vi "MagPowSup.vi"() -> ()   [LabVIEW 2016]
uses:
  <vilib>/Math Plots/3D Math Plots/3D Comet/3D Comet Datatype/3D Comet Datatype.lvclass
  <vilib>/Math Plots/3D Math Plots/3D Comet/3D Comet Datatype/Public/Plot Helper (Vector).vi
  <vilib>/Math Plots/3D Math Plots/3D Comet/3D Comet XCtrl/3D Comet.xctl
panel:
  out "3D Comet":refnum<class "3D Plot Datatype.lvclass">[](xcontrol)
  in  "Z VISA In":refnum<visa-resource-name>="COM3"
  in  "Y VISA In":refnum<visa-resource-name>="COM3"
  out "Z VISA Out":refnum<visa-resource-name>
  out "Y VISA Out":refnum<visa-resource-name>
  out "X VISA Out":refnum<visa-resource-name>
  in  "X VISA In":refnum<visa-resource-name>="COM3"
  in  "Loop":bool
  in  "Loop":bool
  in  "Queue Z":string[][](table)
  in  "Queue Y":string[][](table)
  in  "Queue X":string[][](table)
  in  "Loop":bool
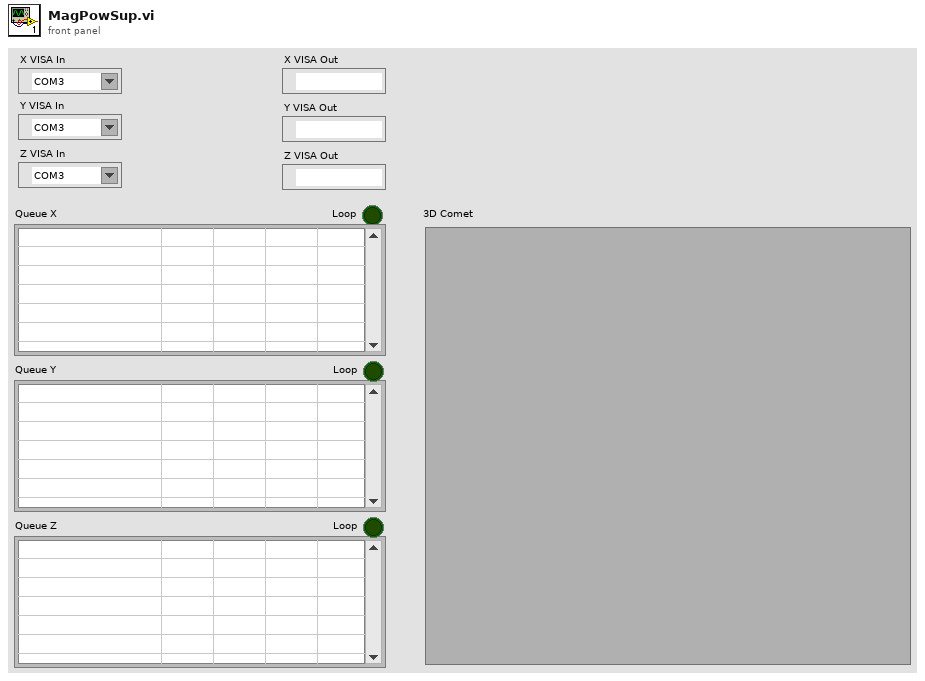
[diagram p1: front panel]
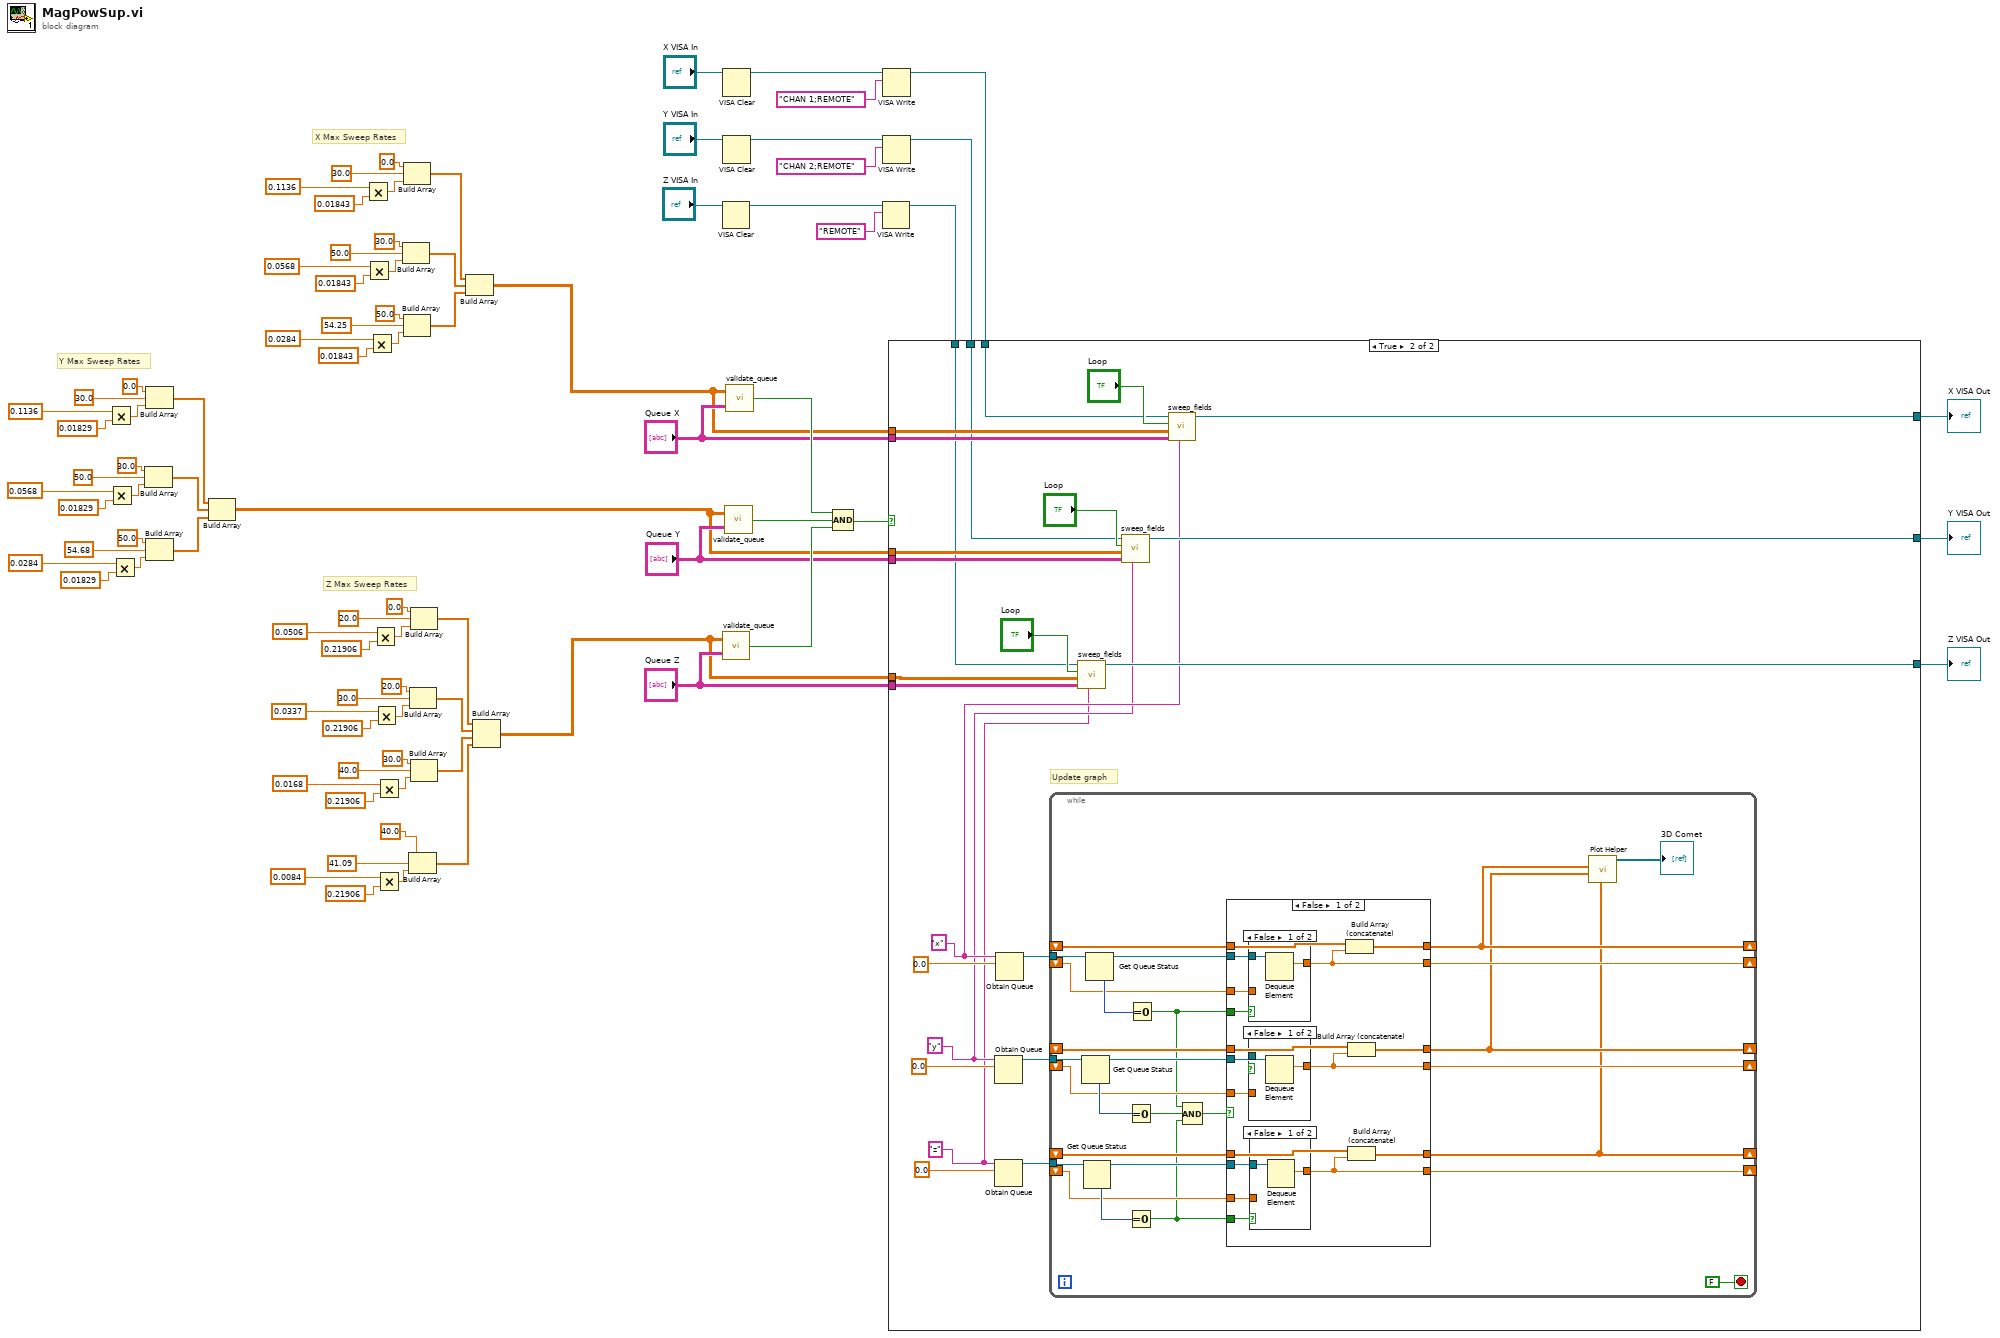
[diagram p0: block diagram]
diagram:
  # "X Max Sweep Rates"
  # "Y Max Sweep Rates"
  # "Z Max Sweep Rates"
  n1 = Multiply(x=0.1136 ("element"), y=0.01829) -> (x*y=w25:dbl)
  n2 = Multiply(x=0.0568 ("element"), y=0.01829) -> (x*y=w23:dbl)
  n3 = Multiply(x=0.0284 ("element"), y=0.01829) -> (x*y=w22:dbl)
  n4 = Build Array(30.0 ("element"), 50.0 ("element"), w23) -> (w31:dbl[])
  n5 = Build Array(0.0 ("element"), 30.0 ("element"), w25) -> (w32:dbl[])
  n6 = Build Array(50.0 ("element"), 54.68 ("element"), w22) -> (w30:dbl[])
  n7 = Build Array(w32, w31, w30) -> (w20:dbl[][])
  n8 = Multiply(x=0.1136 ("element"), y=0.01843) -> (x*y=w6:dbl)
  n9 = Multiply(x=0.0568 ("element"), y=0.01843) -> (x*y=w4:dbl)
  n10 = Multiply(x=0.0284 ("element"), y=0.01843) -> (x*y=w3:dbl)
  n11 = Multiply(x=0.0506 ("element"), y=0.21906) -> (x*y=w65:dbl)
  n12 = Multiply(x=0.0337 ("element"), y=0.21906) -> (x*y=w63:dbl)
  n13 = Multiply(x=0.0168 ("element"), y=0.21906) -> (x*y=w62:dbl)
  n14 = Multiply(x=0.0084 ("element"), y=0.21906) -> (x*y=w60:dbl)
  n15 = Build Array(30.0 ("element"), 50.0 ("element"), w4) -> (w12:dbl[])
  n16 = Build Array(0.0 ("element"), 30.0 ("element"), w6) -> (w13:dbl[])
  n17 = Build Array(50.0 ("element"), 54.25 ("element"), w3) -> (w11:dbl[])
  n18 = Build Array(40.0 ("element"), 41.09 ("element"), w60) -> (w71:dbl[])
  n19 = Build Array(20.0 ("element"), 30.0 ("element"), w63) -> (w73:dbl[])
  n20 = Build Array(0.0 ("element"), 20.0 ("element"), w65) -> (w74:dbl[])
  n21 = Build Array(30.0 ("element"), 40.0 ("element"), w62) -> (w72:dbl[])
  n22 = Build Array(w13, w12, w11) -> (w1:dbl[][])
  n23 = Build Array(w74, w73, w72, w71) -> (w39:dbl[][])
  n24 = VISA Clear(VISA resource name="Z VISA In") -> (VISA resource name out=w42:refnum<visa-resource-name>)  [unwired: 1 in, 1 out]
  n25 = call "validate_queue.vi"("Queue"="Queue Z", "Max Sweep Rates"=w39) -> ("Valid?"=w56:bool)
  n26 = VISA Clear(VISA resource name="X VISA In") -> (VISA resource name out=w84:refnum<visa-resource-name>)  [unwired: 1 in, 1 out]
  n27 = VISA Clear(VISA resource name="Y VISA In") -> (VISA resource name out=w46:refnum<visa-resource-name>)  [unwired: 1 in, 1 out]
  n28 = call "validate_queue.vi"("Queue"="Queue Y", "Max Sweep Rates"=w20) -> ("Valid?"=w57:bool)
  n29 = call "validate_queue.vi"("Queue"="Queue X", "Max Sweep Rates"=w1) -> ("Valid?"=w58:bool)
  n30 = Compound Arithmetic op=AND(w58, w57, w56) -> (w55:bool)
  n31 = VISA Write(VISA resource name=w42, write buffer="REMOTE") -> (VISA resource name out=w40:refnum<visa-resource-name>)  [unwired: 1 in, 2 out]
  n32 = VISA Write(VISA resource name=w84, write buffer="CHAN 1;REMOTE") -> (VISA resource name out=w48:refnum<visa-resource-name>)  [unwired: 1 in, 2 out]
  n33 = VISA Write(VISA resource name=w46, write buffer="CHAN 2;REMOTE") -> (VISA resource name out=w44:refnum<visa-resource-name>)  [unwired: 1 in, 2 out]
  n34 = case shown="True" w55 {
    tunnel: [w86 w112] -> w49
    tunnel: [w87 w111] -> w50
    tunnel: [w88 w110] -> w51
    tunnel: "Queue Y" -> [_ w109]
    tunnel: "Queue X" -> [_ w108]
    tunnel: "Queue Z" -> [_ w107]
    tunnel: w1 -> [_ w106]
    tunnel: w20 -> [_ w105]
    tunnel: w39 -> [_ w104]
    tunnel: w48 -> [w88 w100]
    tunnel: w44 -> [w87 w99]
    tunnel: w40 -> [w86 w98]
    frame False {
    }
    frame True {
      w89 = "z" ("name (unnamed)")
      w90 = "y" ("name (unnamed)")
      w91 = "x" ("name (unnamed)")
      # "Update graph"
      n35 = Obtain Queue(name (unnamed)=w90, element data type=0.0 ("element")) -> (queue out=w92:refnum<queue>)  [unwired: 3 in, 2 out]
      n36 = Obtain Queue(name (unnamed)=w89, element data type=0.0 ("element")) -> (queue out=w93:refnum<queue>)  [unwired: 3 in, 2 out]
      n37 = Obtain Queue(name (unnamed)=w91, element data type=0.0 ("element")) -> (queue out=w94:refnum<queue>)  [unwired: 3 in, 2 out]
      n38 = while {
        tunnel: w94 -> [w134]
        tunnel: w93 -> [w130]
        tunnel: w92 -> [w132]
        shift-right: [w116] -> _
        shift-left: _ -> [w136]
        shift-right: [w115] -> _
        shift-left: _ -> [w137]
        shift-right: [w114] -> _
        shift-left: _ -> [w138]
        shift-right: [w128] -> _
        shift-left: _ -> [w120]
        shift-right: [w127] -> _
        shift-left: _ -> [w121]
        shift-right: [w126] -> _
        shift-left: _ -> [w119]
        stop <- FALSE stop-if-true
        n39 = Get Queue Status(queue=w132) -> (queue out=w133:refnum<queue>, # elements in queue=w125:i32)  [unwired: 2 in, 6 out]
        n40 = Get Queue Status(queue=w130) -> (queue out=w131:refnum<queue>, # elements in queue=w124:i32)  [unwired: 2 in, 6 out]
        n41 = Get Queue Status(queue=w134) -> (queue out=w135:refnum<queue>, # elements in queue=w129:i32)  [unwired: 2 in, 6 out]
        n42 = Equal To 0?(x=w125) -> (x = 0?=w123:bool)
        n43 = Equal To 0?(x=w124) -> (x = 0?=w117:bool)
        n44 = Equal To 0?(x=w129) -> (x = 0?=w118:bool)
        n45 = Compound Arithmetic op=AND(w118, w123, w117) -> (w122:bool)
        n46 = case shown="False" w122 {
          tunnel: [w156 w171] -> w116
          tunnel: [w155 w170] -> w115
          tunnel: [w154 w169] -> w114
          tunnel: w138 -> [w153 w169]
          tunnel: w137 -> [w152 w170]
          tunnel: w136 -> [w151 w171]
          tunnel: w135 -> [w150 _]
          tunnel: w133 -> [w149 _]
          tunnel: w131 -> [w148 _]
          tunnel: [w147 w167] -> w128
          tunnel: [w146 w168] -> w127
          tunnel: [w145 w166] -> w126
          tunnel: w121 -> [w142 w168]
          tunnel: w120 -> [w143 w167]
          tunnel: w119 -> [w140 w166]
          tunnel: w118 -> [w144 _]
          tunnel: w117 -> [w141 _]
          frame False {
            n47 = case shown="False" w144 {
              tunnel: w150 -> [w164 _]
              tunnel: [w163 w165] -> w147
              tunnel: w143 -> [_ w165]
              frame False {
                n48 = Dequeue Element(queue=w164) -> (element=w163:dbl)  [unwired: 2 in, 3 out]
              }
              frame True {
              }
            }
            n49 = case shown="False" {
              selector: _ -> [_ _]
              tunnel: w149 -> [w161 _]
              tunnel: [w160 w162] -> w146
              tunnel: w142 -> [_ w162]
              frame False {
                n50 = Dequeue Element(queue=w161) -> (element=w160:dbl)  [unwired: 2 in, 3 out]
              }
              frame True {
              }
            }
            n51 = case shown="False" w141 {
              tunnel: w148 -> [w158 _]
              tunnel: [w157 w159] -> w145
              tunnel: w140 -> [_ w159]
              frame False {
                n52 = Dequeue Element(queue=w158) -> (element=w157:dbl)  [unwired: 2 in, 3 out]
              }
              frame True {
              }
            }
            n53 = Build Array (concatenate)(w151, w147) -> (w156:dbl[])
            n54 = Build Array (concatenate)(w152, w146) -> (w155:dbl[])
            n55 = Build Array (concatenate)(w153, w145) -> (w154:dbl[])
          }
          frame True {
          }
        }
        n56 = call-poly <vilib>:"Plot Helper.vi"("z vector"=w114, "y vector"=w115, "x vector"=w116) -> ("3D Plot lvclass Array out"=→"3D Comet":refnum<class "3D Plot Datatype.lvclass">[])  [unwired: 3 in, 5 out]
      }
      n57 = call "sweep_fields.vi"("Axis"=w89, "Queue"=w107, "Max Sweep Rates"=w104, "Loop"="Loop", "VISA In"=w98) -> ("VISA Out"=w112:refnum<visa-resource-name>)  [unwired: 6 in]
      n58 = call "sweep_fields.vi"("Axis"=w90, "Queue"=w109, "Max Sweep Rates"=w105, "Loop"="Loop", "VISA In"=w99) -> ("VISA Out"=w111:refnum<visa-resource-name>)  [unwired: 6 in]
      n59 = call "sweep_fields.vi"("Axis"=w91, "Queue"=w108, "Max Sweep Rates"=w106, "Loop"="Loop", "VISA In"=w100) -> ("VISA Out"=w110:refnum<visa-resource-name>)  [unwired: 6 in]
    }
  }
  "X VISA Out" <- w51
  "Y VISA Out" <- w50
  "Z VISA Out" <- w49
